vi "NavigatorInputPrimitive.vi"(0 "error in":errorcluster, 2 "Component":T2 items=["left_itb", "right_itb", "torso_left_itb", "torso_right_itb"], 3 "node":string) -> (1 "error out":errorcluster, 4 "Navigator Inputs":T1)   [LabVIEW 2010]
doc: "This VI gets the status of the Navigator Buttons"
uses:
  <userlib>/ROSforLV_0.1/ROS/Code/SubVIs/BaxterButtons.ctl
panel:
  out "Reply":string
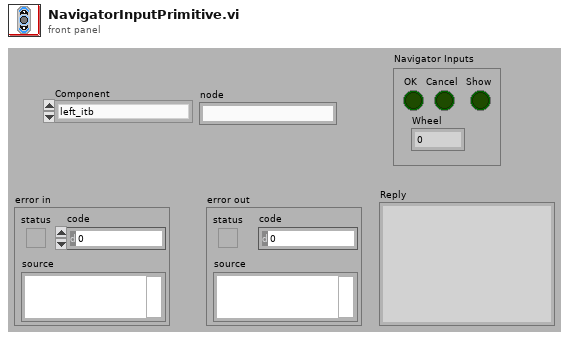
[diagram p1: front panel]
types:
  T1 = cluster{"OK":bool, "Cancel":bool, "Show":bool, "Wheel":u8}
  T2 = typedef "BaxterButtons.ctl" = u16
  T3 = typedef "_ROSControl.ctl" = cluster{"topic port":u16, "Node":string, "topic":string, "type":string, "node port":u32, "error ":errorcluster, "Direction":T4, "APIs":string[]}
  T4 = typedef "_ROSDirection.ctl" = enum16{"Node", "Publisher", "Subscriber", "Service Client"}
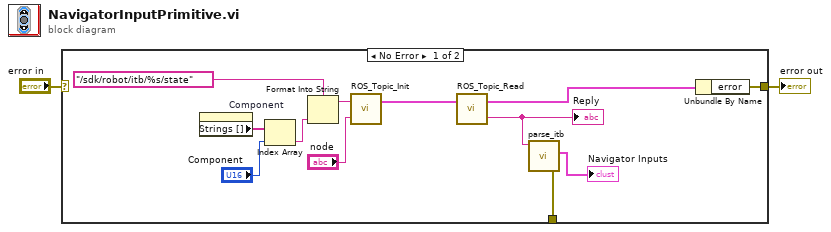
[diagram p0: block diagram]
diagram:
  n1 = case shown="No Error" "error in" {
    selector: "error in" -> [_ w15]
    tunnel: [w14 w15] -> w2
    tunnel: [w3 _] -> _
    frame No Error {
      n2 = property on="Component" class="Ring (strict)"() -> ("Strings []"=w10:string[])  [unwired: 2 in, 2 out]
      n3 = Index Array(array=w10, index="Component") -> (element=w7:string)
      n4 = Format Into String(format string="/sdk/robot/itb/%s/state" ("topic"), w7) -> (resulting string=w6:string)  [unwired: 2 in, 1 out]
      n5 = call <userlib>:"ROS_Topic_Init.vi"("node"="node", "topic"=w6) -> ("ROS out"=w12:T3)  [unwired: 1 in]
      n6 = call <userlib>:"ROS_Topic_Read.vi"("ROS in"=w12) -> ("Reply"=w5:string, "ROS out"=w11:T3)  [unwired: 1 in]
      "Reply" <- w5
      n7 = call <userlib>:"parse_itb.vi"("msg in"=w5) -> ("error out"=w3:errorcluster, "Navigator Inputs"=→"Navigator Inputs":T1)  [unwired: 4 in, 1 out]
      n8 = Unbundle By Name(w11) -> ("error"=w14:errorcluster)
    }
    frame Error {
    }
  }
  "error out" <- w2
